vi "RSNRPZ Get Video Bandwidth List.vi"(8 "error in (no error)":errorcluster, 9 "Buffer Size (200)":i32=200, 10 "Channel (1)":i32=1, 11 "VISA session":refnum<visa-resource-name> caption="VISA resource name") -> (0 "error out":errorcluster, 2 "Bandwidth List":string, 3 "dup VISA session":refnum<visa-resource-name> caption="VISA resource name")   [LabVIEW 2010]
doc: "This VI queries the list of possible video bandwidths.\n\nRemote-control command(s):\nSENSe:BWIDth:VIDeo:LIST?"
uses:
  rsnrpz_32.dll
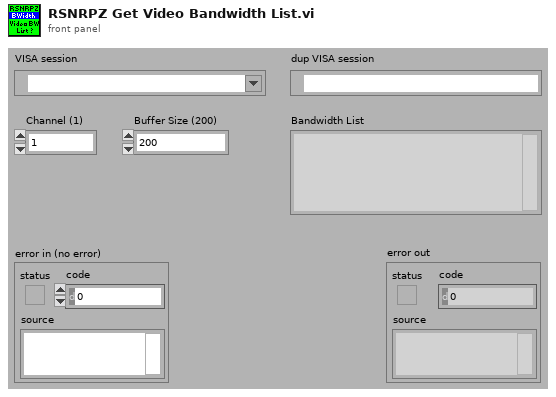
[diagram p1: front panel]
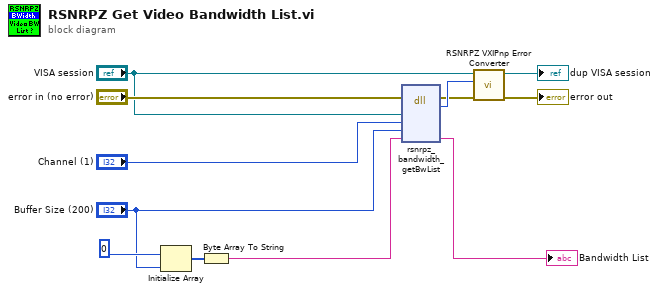
[diagram p0: block diagram]
diagram:
  n1 = Initialize Array(u8 0, "Buffer Size (200)") -> (w11:u8[])
  n2 = Byte Array To String(unsigned byte array=w11) -> (string=w8:string)
  n3 = dll-call lib="rsnrpz_32.dll" fn="rsnrpz_bandwidth_getBwList"(error in="error in (no error)", "Instrument Handle"="VISA session", "Channel"="Channel (1)", "Buffer Size"="Buffer Size (200)", "Bandwidth List"=w8) -> (error out=w5:errorcluster, "Status"=w10:i32, "Bandwidth List"=→"Bandwidth List":string)  [unwired: 5 in, 1 out]
  n4 = call <instrlib>:"RSNRPZ VXIPnp Error Converter.vi"("error in"=w5, "VXIPnp error code"=w10, "VISA session"="VISA session") -> ("error out"=→"error out":errorcluster, "dup VISA session"=→"dup VISA session":refnum<visa-resource-name>)  [unwired: 7 in]
